vi "setPoints.vi"(8 "error in (no error)":errorcluster, 10 "Points":cluster{"X":dbl, "Y":dbl}[](array[cluster]), 11 "Polygon in":refnum<class "Polygon.lvclass">) -> (0 "error out":errorcluster, 3 "Polygon out":refnum<class "Polygon.lvclass">)   [LabVIEW 2013, in "Polygon.lvclass"]
uses:
  Polygon.lvclass
  Polygon.lvclass/Polygon.ctl
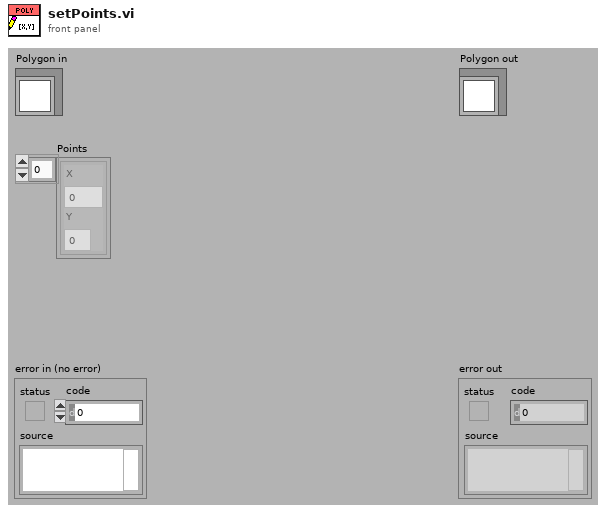
[diagram p1: front panel]
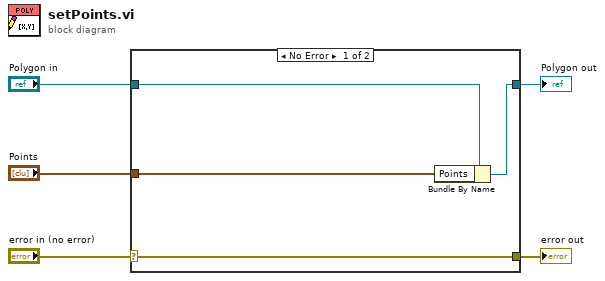
[diagram p0: block diagram]
diagram:
  n1 = case shown="No Error" "error in (no error)" {
    selector: "error in (no error)" -> [w9 w10]
    tunnel: [w9 w10] -> w4
    tunnel: [w7 w11] -> w2
    tunnel: "Polygon in" -> [w8 w11]
    tunnel: "Points" -> [w6 _]
    frame No Error {
      n2 = Bundle By Name(cluster=w8, "Points"=w6) -> (w7:refnum<class "Polygon.lvclass">)
    }
    frame Error {
    }
  }
  "error out" <- w4
  "Polygon out" <- w2
